vi "Conditionally Add SSM Parameter.vi"(10 "create SSM (F)":bool, 11 "parameters in":T1[](array[typedef])) -> (3 "parameters out":T1[](array[typedef]))   [LabVIEW 2020]
uses:
  VS Channel Definition for Parameter.ctl
  Parameter Definition.ctl
  <vilib>/NI/NI VeriStand Encoding and Decoding/Encoding.ctl
  <vilib>/NI/NI VeriStand Encoding and Decoding/Encoding and Decoding.lvlib
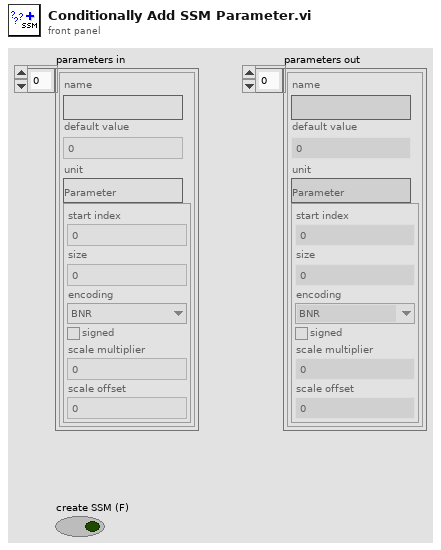
[diagram p1: front panel]
types:
  T1 = typedef "VS Channel Definition for Parameter.ctl" = cluster{"name":string, "default value":dbl, "unit":string, "Parameter":T2}
  T2 = typedef "Parameter Definition.ctl" = cluster{"start index":i32, "size":i32, "encoding":T3, "signed":bool, "scale multiplier":dbl, "scale offset":dbl}
  T3 = typedef "Encoding and Decoding.lvlib/Encoding.ctl" = enum16{"BNR", "BCD", "Discrete"}
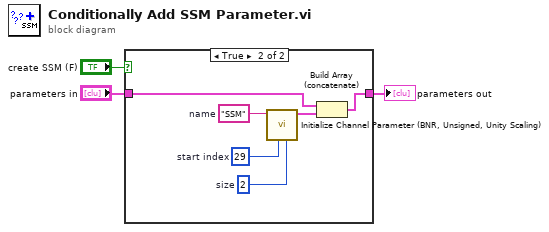
[diagram p0: block diagram]
diagram:
  n1 = case shown="True" "create SSM (F)" {
    tunnel: "parameters in" -> [w4 w10]
    tunnel: [w4 w9] -> w3
    frame False {
    }
    frame True {
      w6 = 2  # size
      w7 = 29  # start index
      w8 = "SSM"  # name
      n2 = call "Initialize Channel Parameter (BNR, Unsigned, Unity Scaling).vi"("size"=w6, "start index"=w7, "name"=w8) -> ("channel parameter"=w5:T1)  [unwired: 8 in]
      n3 = Build Array (concatenate)(w10, w5) -> (w9:T1[])
    }
  }
  "parameters out" <- w3
